vi "MListbox Insert Rows.vi"(8 "error in (no error)":errorcluster, 9 "Rows":string[][](array[string]), 10 "Index":i16=-1, 11 "Multicolumn ListBox in":refnum<class "Multicolumn ListBox.lvclass">) -> (0 "error out":errorcluster, 3 "Multicolumn ListBox out":refnum<class "Multicolumn ListBox.lvclass">)   [LabVIEW 2018, in "Multicolumn ListBox.lvclass"]
uses:
  Multicolumn ListBox.lvclass
  Multicolumn ListBox.lvclass/Multicolumn ListBox.ctl
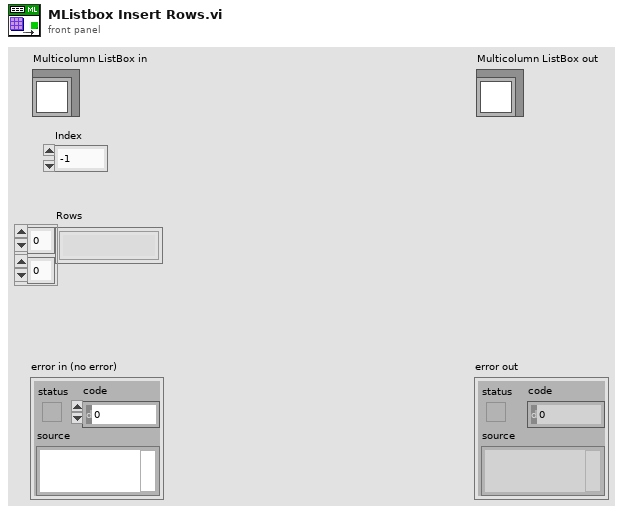
[diagram p1: front panel]
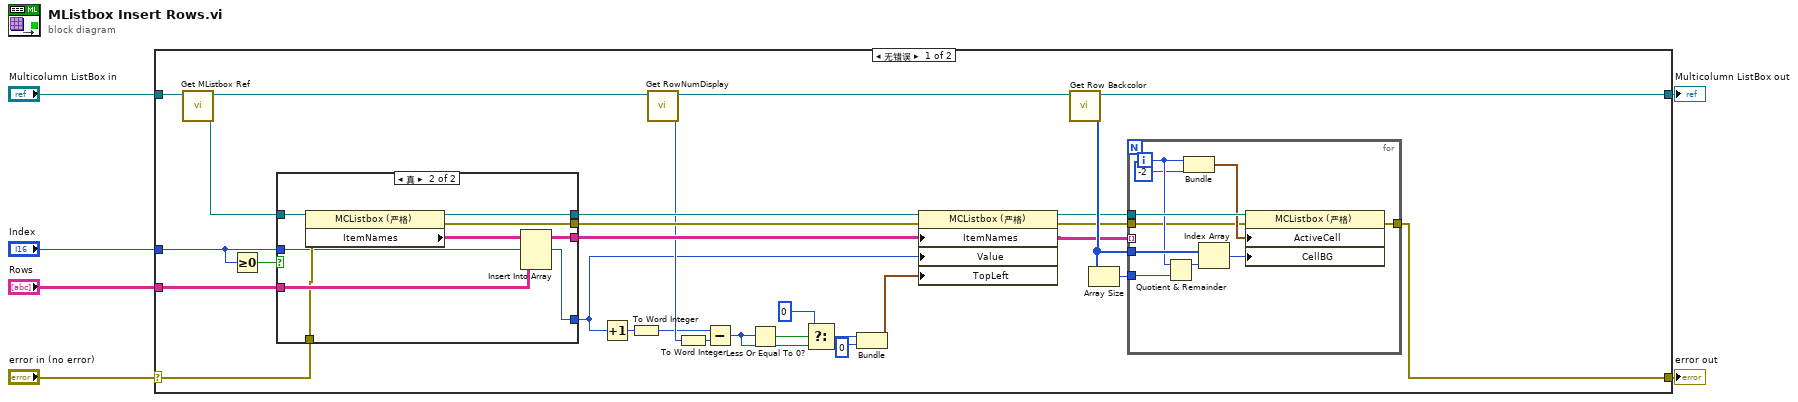
[diagram p0: block diagram]
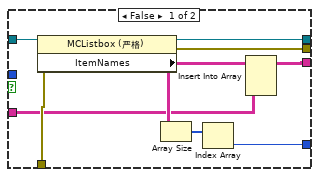
[diagram p2: hidden frame]
diagram:
  n1 = case shown="无错误" "error in (no error)" {
    selector: "error in (no error)" -> [w29 w63]
    tunnel: [w7 w63] -> w5
    tunnel: [w8 w62] -> w3
    tunnel: "Multicolumn ListBox in" -> [w34 w62]
    tunnel: "Index" -> [w19 _]
    tunnel: "Rows" -> [w32 _]
    frame No Error {
      n2 = call "Get MListbox Ref.vi"("Multicolumn ListBox in"=w34) -> ("MListbox Ref"=w33:refnum<vi>, "Multicolumn ListBox out"=w30:refnum<class "Multicolumn ListBox.lvclass">)  [unwired: 8 in, 1 out]
      n3 = Greater Or Equal To 0?(x=w19) -> (x >= 0?=w20:bool)
      n4 = case shown="真" w20 {
        tunnel: w33 -> [w43 w51]
        tunnel: w32 -> [w37 w49]
        tunnel: w29 -> [w41 w48]
        tunnel: [w42 w47] -> w28
        tunnel: [w36 w46] -> w26
        tunnel: [w35 w45] -> w25
        tunnel: w19 -> [_ w44]
        tunnel: [w39 w44] -> w10
        frame False {
          n5 = property class="MCListbox (严格)"(reference=w43, error in=w41) -> (reference out=w42:refnum<vi>, error out=w35:errorcluster, "ItemNames"=w38:string[][])
          n6 = Array Size(array=w38) -> (size(s)=w40:i32[])
          n7 = Index Array(array=w40) -> (element=w39:i32)  [unwired: 1 in]
          n8 = Insert Into Array(array=w38, new element=w37) -> (w36:string[][])  [unwired: 2 in]
        }
        frame True {
          n9 = property class="MCListbox (严格)"(reference=w51, error in=w48) -> (reference out=w47:refnum<vi>, error out=w45:errorcluster, "ItemNames"=w50:string[][])
          n10 = Insert Into Array(array=w50, index (row)=w44, new element=w49) -> (w46:string[][])  [unwired: 1 in]
        }
      }
      n11 = Increment(x=w10) -> (x+1=w21:i32)
      n12 = To Word Integer(number=w21) -> (16bit integer=w9:i16)
      n13 = call "Get RowNumDisplay.vi"("Multicolumn ListBox in"=w30) -> ("RowNumDisplay"=w11:u16, "Multicolumn ListBox out"=w22:refnum<class "Multicolumn ListBox.lvclass">)  [unwired: 8 in, 1 out]
      n14 = To Word Integer(number=w11) -> (16bit integer=w13:i16)
      n15 = Subtract(x=w9, y=w13) -> (x-y=w16:i16)
      n16 = Less Or Equal To 0?(x=w16) -> (x <= 0?=w18:bool)
      n17 = Select(t=0, s=w18, f=w16) -> (s? t:f=w15:i32)
      n18 = Bundle(w15, 0) -> (w12:cluster{i32, i32})  [unwired: 1 in]
      n19 = property class="MCListbox (严格)"(reference=w28, error in=w25, "ItemNames"=w26, "Value"=w10, "TopLeft"=w12) -> (reference out=w27:refnum<vi>, error out=w24:errorcluster)
      n20 = call "Get Row Backcolor.vi"("Multicolumn ListBox in"=w22) -> ("Row Backcolor"=w31:u32[], "Multicolumn ListBox out"=w8:refnum<class "Multicolumn ListBox.lvclass">)  [unwired: 8 in, 1 out]
      n21 = Array Size(array=w31) -> (size(s)=w23:i32)
      n22 = for {
        tunnel: w26 -> [_] mode=indexing
        tunnel: w27 -> [w58]
        tunnel: w23 -> [w61]
        tunnel: w31 -> [w60]
        tunnel: w24 -> [w54]
        tunnel: [w52] -> w7
        i -> [w57]
        n23 = Quotient & Remainder(x=w57, y=w61) -> (x-y*floor(x/y)=w59:i32)  [unwired: 1 out]
        n24 = Bundle(w57, "Column"=-2) -> (w55:cluster{i32, "Column":i32})  [unwired: 1 in]
        n25 = Index Array(array=w60, index=w59) -> (element=w53:u32)
        n26 = property class="MCListbox (严格)"(reference=w58, error in=w54, "ActiveCell"=w55, "CellBG"=w53) -> (error out=w52:errorcluster)  [unwired: 1 out]
      }
    }
    frame Error {
    }
  }
  "error out" <- w5
  "Multicolumn ListBox out" <- w3
